vi "test19-1ToNInterruptStatus.vi"(8 "error in (no error)":errorcluster, 11 "TestCase in":refnum<class "testcase-CSMBroadcast.lvclass">) -> (0 "error out":errorcluster, 3 "TestCase out":refnum<class "testcase-CSMBroadcast.lvclass">)   [LabVIEW 2017, in "testcase-CSMBroadcast.lvclass"]
uses:
  testcase-CSMBroadcast.lvclass
  0b17d103-e67b-41be-a9eb-a2ee1311ff1f.vi
  5999693e-4f8a-4b34-ae87-f34dff5771be.vi
  src/user.lib/_NEVSTOP/Communicable State Machine(CSM)/AdvanceAPI/CSM - Get Module Attribute.vi
  <vilib>/addons/_JKI Toolkits/VI Tester/TestCase.llb/TestCase.lvclass
  src/user.lib/_NEVSTOP/Communicable State Machine(CSM)/Communicable State Machine.lvlib
  CSM/CSM-Testcase.lvlib
  C:/Program Files (x86)/National Instruments/LabVIEW 2017/vi.lib/addons/_JKI Toolkits/VI Tester/TestCase.llb/TestCase.lvclass
panel:
  out "LoopCount2":i32
  out "LoopCount":i32
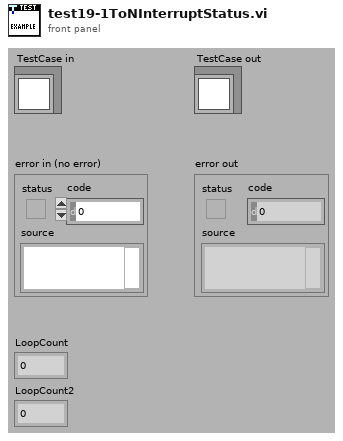
[diagram p1: front panel]
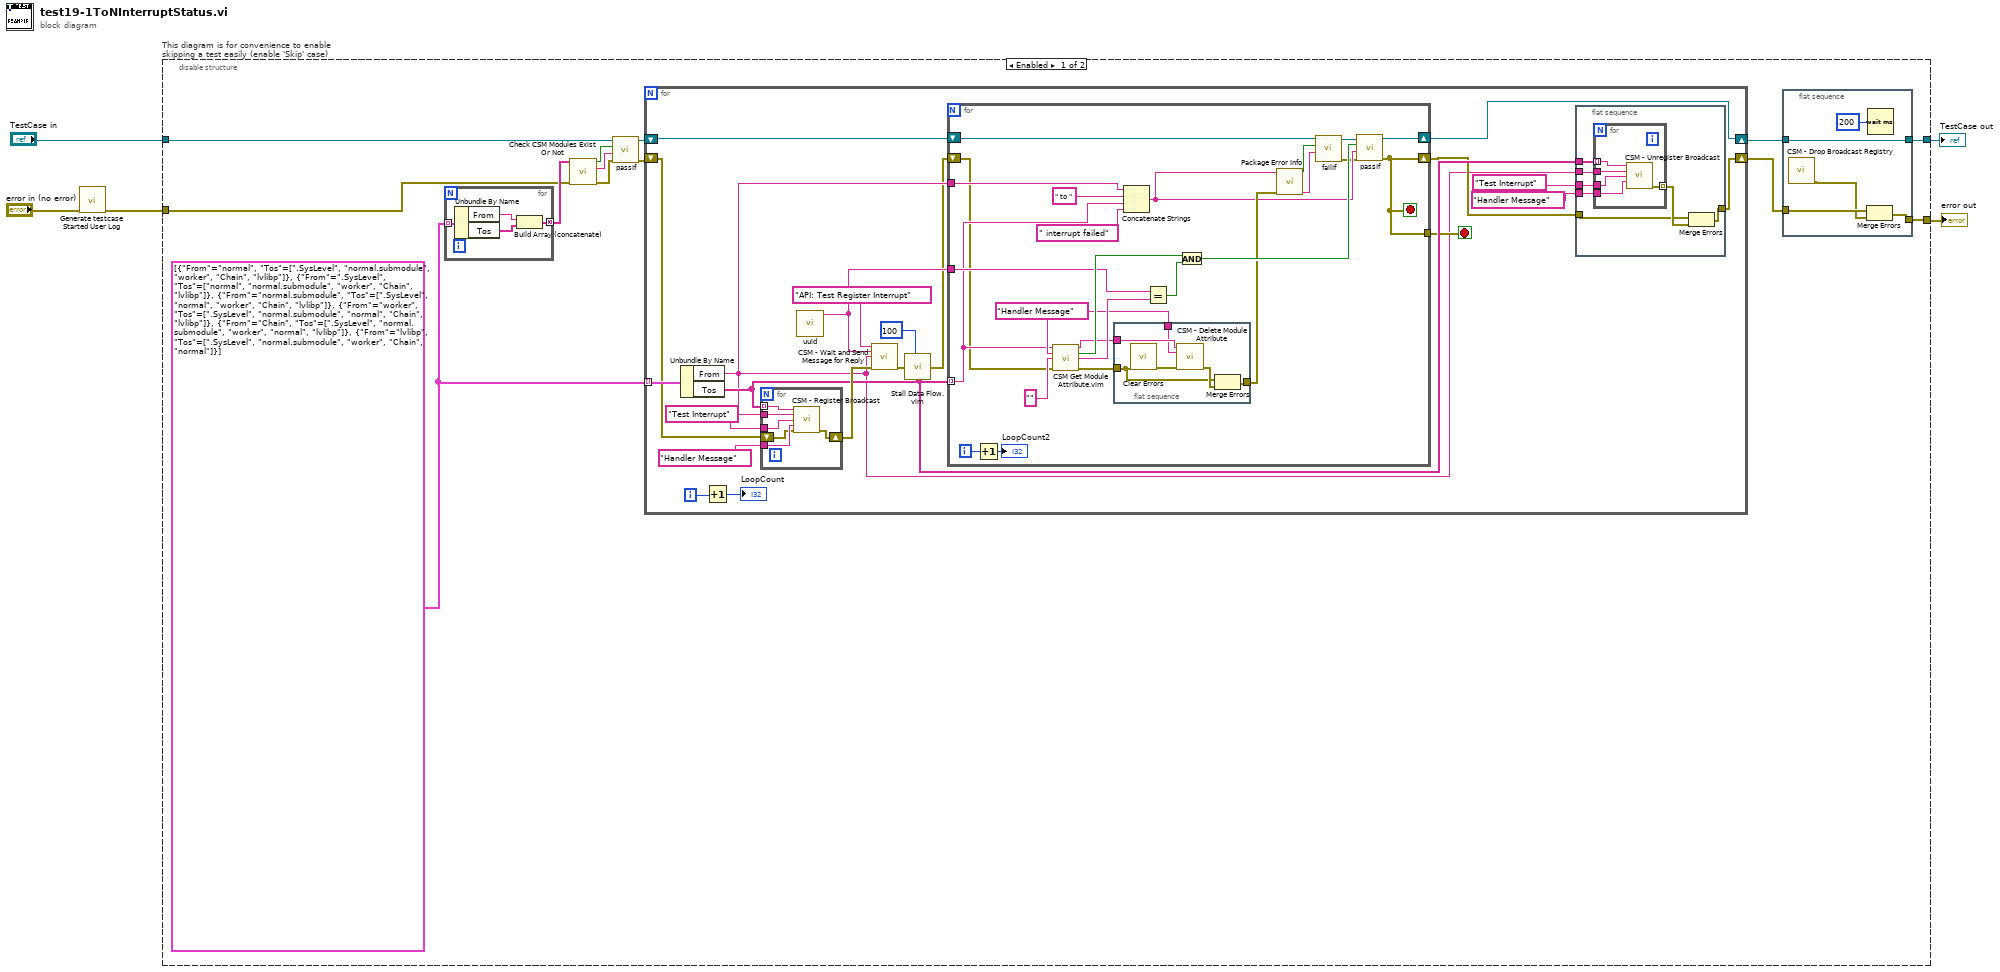
[diagram p0: block diagram]
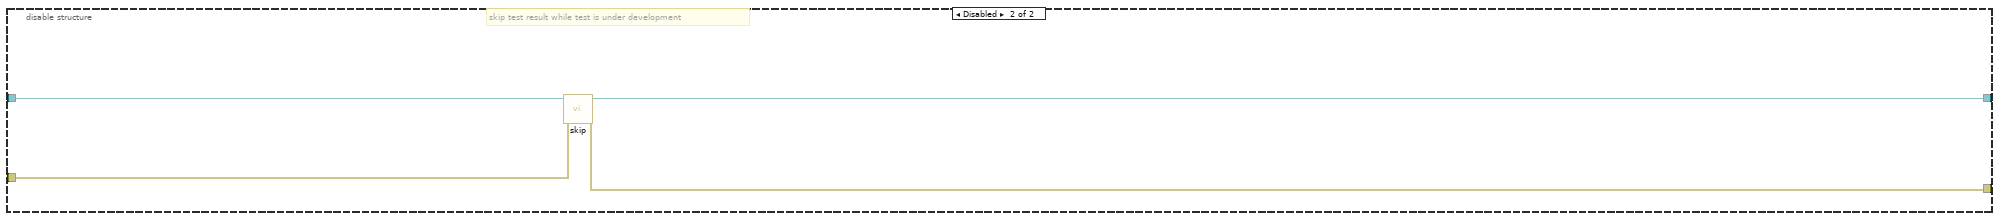
[diagram p2: hidden frame]
diagram:
  n1 = call "Generate testcase Started User Log.vi"("Error In"="error in (no error)") -> ("error out"=w1:errorcluster)  [unwired: 10 in]
  n2 = disable-structure "This diagram is for convenience to enable skipping a test easily (enable 'Skip' case)" shown="Enabled" {
    disable-tunnel: "TestCase in" -> [w11 w101]
    disable-tunnel: [w6 w99] -> w2
    disable-tunnel: [w17 w100] -> w4
    disable-tunnel: w1 -> [w8 w98]
    frame Enabled {
      w12 = cluster{"From":string, "Tos":string[]}[] [{"From"="normal", "Tos"=[".SysLevel", "normal.submodule", "worker", "Chain", "lvlibp"]}, {"From"=".SysLevel", "Tos"=["normal", "normal.submodule", "worker", "Chain", "lvlibp"]}, {"From"="normal.submodule", "Tos"=[".SysLevel", "normal", "worker", "Chain", "lvlibp"]}, {"From"="worker", "Tos"=[".SysLevel", "normal.submodule", "normal", "Chain", "lvlibp"]}, {"From"="Chain", "Tos"=[".SysLevel", "normal.submodule", "worker", "normal", "lvlibp"]}, {"From"="lvlibp", "Tos"=[".SysLevel", "normal.submodule", "worker", "Chain", "normal"]}]
      n3 = for {
        tunnel: w12 -> [w22] mode=indexing
        tunnel: [w19] -> w13 mode=concatenating
        n4 = Unbundle By Name(w22) -> ("From"=w21:string, "Tos"=w20:string[])
        n5 = Build Array (concatenate)(w21, w20) -> (w19:string[])
      }
      n6 = call "Check CSM Modules Exist Or Not.vi"("error in"=w8, "CSM names in"=w13) -> ("error out"=w14:errorcluster, "Debug string"=w15:string, "All Modules Exist?"=w16:bool)  [unwired: 7 in]
      n7 = call-dynamic "passIf.vi"("error in (no error)"=w14, "message (\"\")"=w15, "pass"=w16, "TestCase in"=w11) -> ("error out"=w9:errorcluster, "TestCase out"=w10:refnum<class "testcase-CSMBroadcast.lvclass">)  [unwired: 6 in]
      n8 = for {
        shift-right: [w37] -> w18
        shift-left: w9 -> [w29]
        shift-right: [w33] -> w7
        shift-left: w10 -> [w41]
        tunnel: w12 -> [w46] mode=indexing
        i -> [w48]
        stop <- w32 stop-if-true
        n9 = Unbundle By Name(w46) -> ("From"=w30:string, "Tos"=w36:string[])
        n10 = Increment(x=w48) -> (x+1=→"LoopCount":i32)
        n11 = for {
          tunnel: w30 -> [w97]
          tunnel: w36 -> [w96] mode=indexing
          tunnel: "Test Interrupt" -> [w95]
          tunnel: "Handler Message" -> [w94]
          shift-right: [w93] -> w38
          shift-left: w29 -> [w92]
          n12 = call "CSM - Register Broadcast.vi"("CSM Name(Empty for Broadcast Event)"=w96, "Source CSM Name (* as Default)"=w97, "Trigger"=w95, "API (If \"\", Same as Trigger)"=w94, "Error In"=w92) -> ("error out"=w93:errorcluster)  [unwired: 9 in, 1 out]
        }
        n13 = call "uuid.vi"() -> ("UUID"=w42:string)  [unwired: 11 in]
        n14 = call "CSM - Wait and Send Message for Reply.vi"("State"="API: Test Register Interrupt", "Arguments (\"\")"=w42, "Target Module"=w30, "Error In (No Error)"=w38) -> ("error out"=w44:errorcluster)  [unwired: 8 in, 3 out]
        n15 = call "Stall Data Flow.vim"("value in"=w44, "milliseconds to wait"=u32 100) -> ("value out"=w28:errorcluster)  [unwired: 1 out]
        n16 = for {
          tunnel: w42 -> [w83]
          shift-right: [w81] -> w33
          shift-left: w41 -> [w64]
          shift-right: [w73] -> w31
          shift-left: w28 -> [w61]
          tunnel: w36 -> [w66] mode=indexing
          tunnel: [w73] -> w32
          tunnel: w30 -> [w67]
          i -> [w75]
          stop <- w73 stop-if-true
          w76 = "Handler Message" ("To")
          n17 = Increment(x=w75) -> (x+1=→"LoopCount2":i32)
          n18 = call "CSM Get Module Attribute.vim"("CSM Name"=w66, "Attribute"=w76, "Default Value (Empty Variant)"="", "Error In"=w61) -> ("CSM Name (Dup)"=w77:string, "Found"=w85:bool, "Value"=w82:string, "error out"=w78:errorcluster)  [unwired: 7 in, 1 out]
          n19 = flat-sequence {
            tunnel: w78 -> [w87]
            tunnel: w77 -> [w90]
            tunnel: w76 -> [w89]
            tunnel: [w86] -> w70
            frame #0 {
              n20 = call <vilib>:"Clear Errors.vi"("error in (no error)"=w87) -> ("error out"=w91:errorcluster)  [unwired: 5 in, 1 out]
              n21 = call "CSM - Delete Module Attribute.vi"("CSM Name"=w90, "Attribute"=w89, "Error In"=w91) -> ("error out"=w88:errorcluster)  [unwired: 9 in, 3 out]
              n22 = Merge Errors(w87, w88) -> (w86:errorcluster)
            }
          }
          n23 = Concatenate Strings(w67, " to " ("string"), w66, " interrupt failed" ("string")) -> (w65:string)
          n24 = Equal?(x=w83, y=w82) -> (x = y?=w80:bool)
          n25 = And(x=w85, y=w80) -> (x .and. y?=w79:bool)
          n26 = call "Package Error Info.vi"("error in"=w70, "String in"=w65) -> ("packed error info out"=w71:string, "error status"=w72:bool)  [unwired: 8 in]
          n27 = call-dynamic "failIf.vi"("message (\"\")"=w71, "fail"=w72, "TestCase in"=w64) -> ("error out"=w62:errorcluster, "TestCase out"=w63:refnum<class "testcase-CSMBroadcast.lvclass">)  [unwired: 7 in]
          n28 = call-dynamic "passIf.vi"("error in (no error)"=w62, "message (\"\")"=w65, "pass"=w79, "TestCase in"=w63) -> ("error out"=w73:errorcluster, "TestCase out"=w81:refnum<class "testcase-CSMBroadcast.lvclass">)  [unwired: 6 in]
        }
        n29 = flat-sequence {
          tunnel: [w55] -> w37
          tunnel: w36 -> [w54]
          tunnel: w30 -> [w53]
          tunnel: "Test Interrupt" -> [w52]
          tunnel: "Handler Message" -> [w50]
          tunnel: w31 -> [w49]
          frame #0 {
            n30 = for {
              tunnel: w54 -> [w60] mode=indexing
              tunnel: w53 -> [w59]
              tunnel: w52 -> [w58]
              tunnel: [w57] -> w51 mode=indexing
              tunnel: w50 -> [w56]
              n31 = call "CSM - Unregister Broadcast.vi"("CSM Name(Empty for Broadcast Event)"=w60, "Source CSM Name (* as Default)"=w59, "Trigger"=w58, "API (\"*\" as Default)"=w56) -> ("error out"=w57:errorcluster)  [unwired: 10 in, 1 out]
            }
            n32 = Merge Errors(w49, w51) -> (w55:errorcluster)
          }
        }
      }
      n33 = flat-sequence {
        tunnel: [w27] -> w17
        tunnel: w18 -> [w26]
        tunnel: w7 -> [w24]
        tunnel: [w24] -> w6
        frame #0 {
          n34 = call "CSM - Drop Broadcast Registry.vi"() -> ("error out"=w25:errorcluster)  [unwired: 15 in]
          n35 = Merge Errors(w26, w25) -> (w27:errorcluster)
          n36 = Wait (ms)(milliseconds to wait=u32 200) -> ()  [unwired: 1 out]
        }
      }
    }
    frame Disabled {
      # "skip test result while test is under development"
      n37 = call <vilib>:"skip.vi"("error in (no error)"=w98, "TestCase in"=w101) -> ("error out"=w100:errorcluster, "TestCase out"=w99:refnum<class "testcase-CSMBroadcast.lvclass">)  [unwired: 8 in]
    }
  }
  "error out" <- w4
  "TestCase out" <- w2
